vi "init_prev.vi"(8 "error in (no error)":errorcluster) -> (0 "error out":errorcluster, 3 "output cluster":T1)   [LabVIEW 2025]
uses:
  Classes/Thermocouples/Thermocouples.lvclass
  Classes/Relays/Relays.lvclass
  <vilib>/Utility/sysdir.llb/System Directory Type.ctl
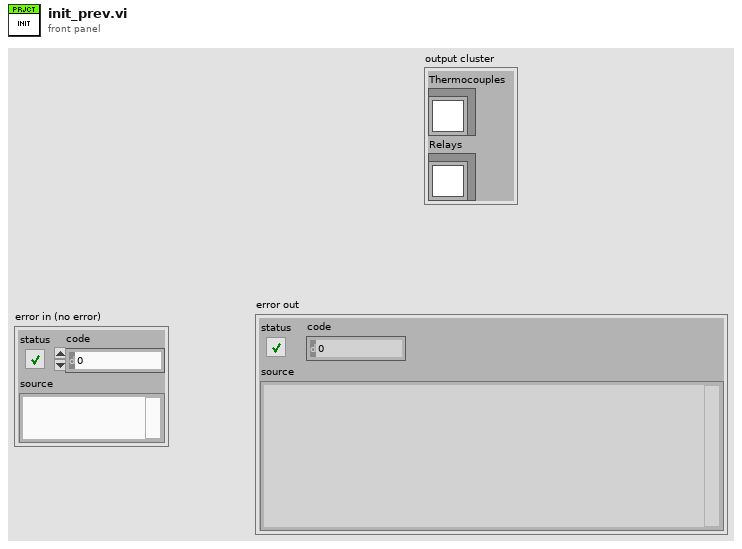
[diagram p1: front panel]
types:
  T1 = cluster{"Thermocouples":refnum<class "Thermocouples.lvclass">, "Relays":refnum<class "Relays.lvclass">}
  T2 = typedef "System Directory Type.ctl" = i32
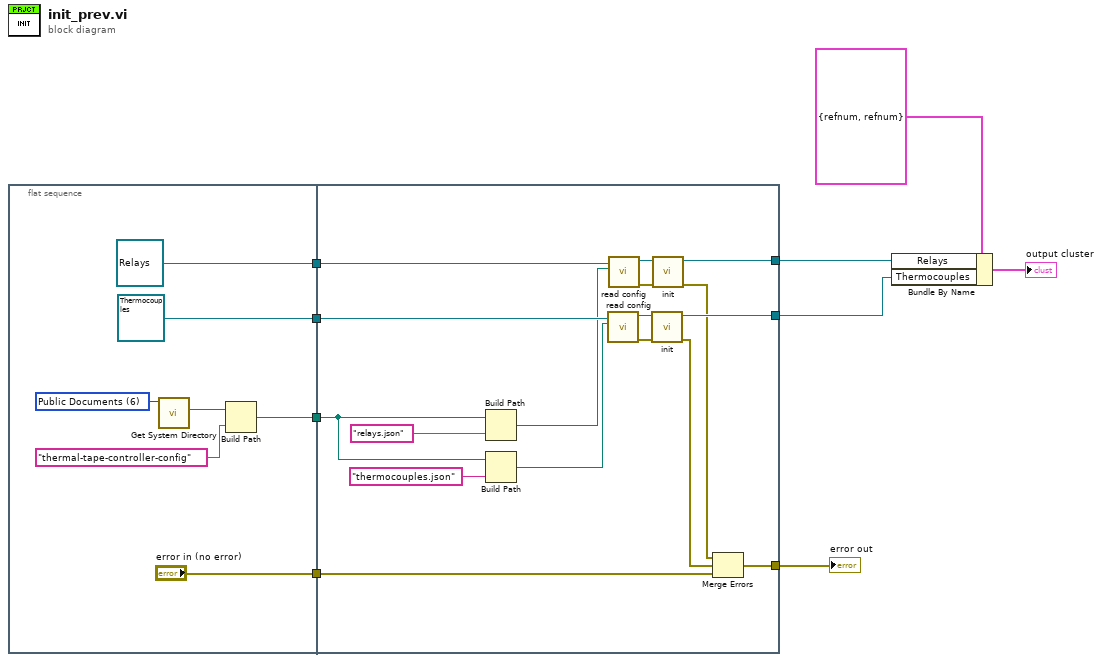
[diagram p0: block diagram]
diagram:
  n1 = flat-sequence {
    tunnel: [refnum<class "Relays.lvclass"> refnum ("Relays.lvclass")] -> w7
    tunnel: [refnum<class "Thermocouples.lvclass"> refnum ("Thermocouples.lvclass")] -> w6
    tunnel: [w13] -> w3
    tunnel: ["error in (no error)"] -> w2
    tunnel: w7 -> [w28]
    tunnel: w6 -> [w29]
    tunnel: [w27] -> w5
    tunnel: [w26] -> w4
    tunnel: w3 -> [w24]
    tunnel: w2 -> [w18]
    tunnel: [w17] -> w1
    frame #0 {
      w16 = T2 6 items=["User Home"=0, "User Desktop"=1, "User Documents"=2, "User Application Data"=3, "User Preferences"=4, "User Temporary"=5, "Public Documents"=6, "Public Application Data"=7, "Public Preferences"=8, "Public Cache"=13, "System Core Libraries"=9, "System Installed Libraries"=10, "Application Files"=11, "Boot Volume Root"=12] ("system directory type")
      n2 = call <vilib>:"Get System Directory.vi"("system directory type"=w16) -> ("system directory"=w15:path)  [unwired: 10 in]
      n3 = Build Path(base path=w15, name or relative path="thermal-tape-controller-config") -> (appended path=w13:path)
    }
    frame #1 {
      n4 = Build Path(base path=w24, name or relative path="relays.json") -> (appended path=w22:path)
      n5 = Build Path(base path=w24, name or relative path="thermocouples.json") -> (appended path=w21:path)
      n6 = call-dynamic "read config.vi"("config file path"=w21, "Processor in"=w29) -> ("error out"=w32:errorcluster, "Processor out"=w33:refnum<class "Thermocouples.lvclass">)  [unwired: 8 in]
      n7 = call-dynamic "read config.vi"("config file path"=w22, "Processor in"=w28) -> ("error out"=w31:errorcluster, "Processor out"=w30:refnum<class "Relays.lvclass">)  [unwired: 8 in]
      n8 = call-dynamic "init.vi"("error in (no error)"=w32, "Thermocouples in"=w33) -> ("error out"=w19:errorcluster, "Thermocouples out"=w27:refnum<class "Thermocouples.lvclass">)  [unwired: 8 in]
      n9 = call-dynamic "init.vi"("error in (no error)"=w31, "Relays in"=w30) -> ("error out"=w20:errorcluster, "Relays out"=w26:refnum<class "Relays.lvclass">)  [unwired: 8 in]
      n10 = Merge Errors(w20, w19, w18) -> (w17:errorcluster)
    }
  }
  n11 = Bundle By Name(cluster=T1 {"Thermocouples"=refnum, "Relays"=refnum}, "Relays"=w4, "Thermocouples"=w5) -> (→"output cluster":T1)
  "error out" <- w1
